vi "testDataAnalog_getIndices.vi"(4 "input_Increment":i32, 6 "input_Total":i32, 7 "input_count":i32) -> (2 "output_increment":i32, 3 "output_IndexStart":i32)   [LabVIEW 2014]
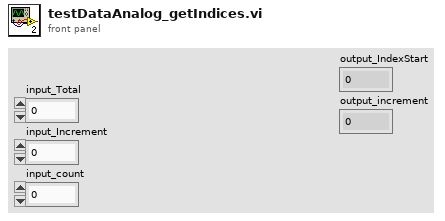
[diagram p1: front panel]
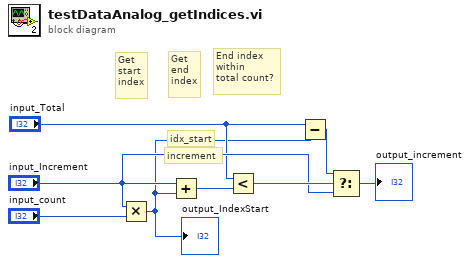
[diagram p0: block diagram]
diagram:
  # "increment"
  # "idx_start"
  # "End index\nwithin\ntotal count?"
  # "Get\nend\nindex"
  # "Get\nstart\nindex"
  n1 = Multiply(x="input_Increment", y="input_count") -> (x*y=w3:i32)
  "output_IndexStart" <- w3
  n2 = Add(x="input_Increment", y=w3) -> (x+y=w7:i32)
  n3 = Less?(x="input_Total", y=w7) -> (x < y?=w6:bool)
  n4 = Subtract(x="input_Total", y=w3) -> (x-y=w2:i32)
  n5 = Select(t=w2, s=w6, f="input_Increment") -> (s? t:f=→"output_increment":i32)
